vi "AgilentDMM.vi"(4 "error in":T15, 7 "Command":T16) -> (0 "error out":T15, 3 "Response":T13)   [LabVIEW 2018]
uses:
  MOKO_LabViewLibrary/MokoLowLevel/MokoLowLovelControl/MLLC_Command.ctl
  MOKO_LabViewLibrary/MokoLowLevel/MokoLowLovelControl/MLLC_Error.ctl
  MOKO_LabViewLibrary/MokoLowLevel/MokoLowLovelControl/MLLC_Mode.ctl
  MOKO_LabViewLibrary/MokoLowLevel/MokoLowLovelControl/MLLC_Response.ctl
  MOKO_LabViewLibrary/MokoLowLevel/MokoLowLovelControl/MLLC_DriverName.ctl
  MOKO_LabViewLibrary/MokoLowLevel/MokoLowLovelControl/MLLC_Request.ctl
  MOKO_LabViewLibrary/MokoLowLevel/MokoLowLovelControl/MLLC_ErrorCode.ctl
  MOKO_LabViewLibrary/MokoLowLevel/MokoLowLovelControl/MLLC_ResponseInit.ctl
  MOKO_LabViewLibrary/MokoLowLevel/MokoLowLovelControl/MLLC_ConnectCluster.ctl
  MOKO_LabViewLibrary/MokoLowLevel/MokoLowLovelControl/MLLC_InterfaceType.ctl
  MOKO_LabViewLibrary/MokoLowLevel/MokoLowLovelControl/MLLC_OpenedSession.ctl
  MOKO_LabViewLibrary/MokoLowLevel/MokoLowLovelControl/MLLC_InterfaceSettings.ctl
  MOKO_LabViewLibrary/MokoLowLevel/MokoLowLovelControl/MLLC_InterfaceKind.ctl
  data/AgilentDMM_Functions.ctl
  data/AgilentDMM_Models.ctl
panel:
  in  "Settings":T9={"Saved Data"=variant, "Permanent data"={"Connect"={"InterfaceType"=enum."VISA", "OpenedSession"="", "InterfaceSettings"={"Interface"=enum."GPIB", "EOS 4 read"=enum."LF (\\n)", "EOS 4 write"=enum."LF (\\n)", "TMO, ms"=5000, "Sett"=variant(cluster{"Baud Rate":u32, "Data Bits":u16, "Parity":u16, "Stop Bits":u16, "Flow Control":u16, "Eho":bool} {"Baud Rate"=75, "Data Bits"=0, "Parity"=0, "Stop Bits"=0, "Flow Control"=0, "Eho"=FALSE})}}, "Channel"=1, "Func"=enum."VDC", "Model"=enum."L4411"}}
  in  "Response Init array":T10[](array[typedef])=["34401", "34405", "34410", "34411", "34420", "34450", "34461", "34465", "34470", "34475", "U2741"]
  in  "Error Code":T6=5475
  in  "Request":T11="*idn?"
  in  "Driver Name":T12="AgilentDMM"
  in  "Mode":T14=enum."Check"
  # "AgilentDMM"
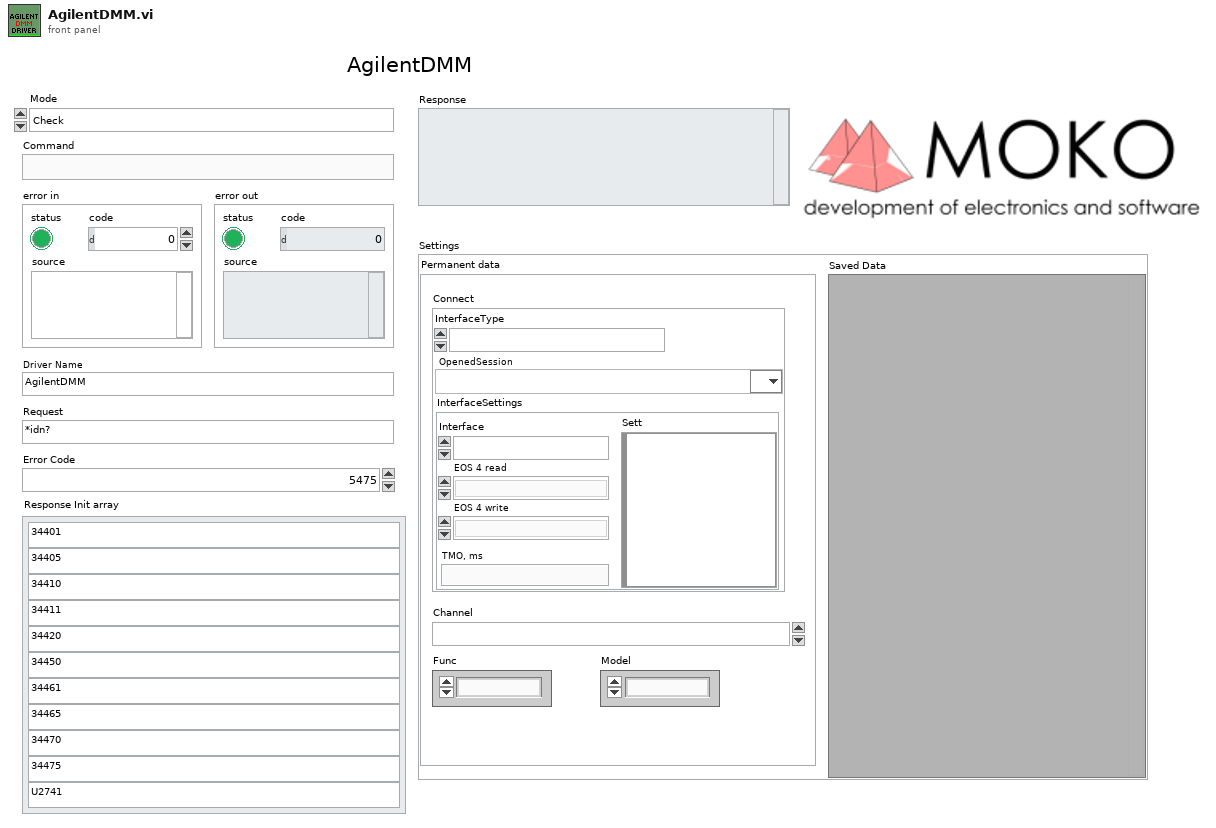
[diagram p1: front panel]
types:
  T1 = typedef "MLLC_ConnectCluster.ctl" = cluster{"InterfaceType":T2, "OpenedSession":T3, "InterfaceSettings":T4}
  T2 = typedef "MLLC_InterfaceType.ctl" = enum16{"VISA", "Prologix USB-GPIB"}
  T3 = typedef "MLLC_OpenedSession.ctl" = refnum<visa-resource-name>
  T4 = typedef "MLLC_InterfaceSettings.ctl" = cluster{"Interface":T5, "EOS 4 read":enum16{"Default (=EOS 4 write)", "CR (\\r)", "LF (\\n)", "None"}, "EOS 4 write":enum16{"CR+LF (\\r\\n)", "CR (\\r)", "LF (\\n)", "None"}, "TMO, ms":i32, "Sett":variant}
  T5 = typedef "MLLC_InterfaceKind.ctl" = enum16{"RS232", "GPIB", "USB", "Ethernet", "another"}
  T6 = typedef "MLLC_ErrorCode.ctl" = u32
  T7 = typedef "AgilentDMM_Functions.ctl" = enum16{"VDC", "VAC", "IDC", "IAC", "F", "R2", "R4", "CAP"}
  T8 = typedef "AgilentDMM_Models.ctl" = enum16{"34401", "34461", "34410", "34411", "34420", "34450", "34405", "U2741", "34470", "34465", "34460", "L4411"}
  T9 = cluster{"Saved Data":variant, "Permanent data":cluster{"Connect":T1, "Channel":T6, "Func":T7, "Model":T8}}
  T10 = typedef "MLLC_ResponseInit.ctl" = string
  T11 = typedef "MLLC_Request.ctl" = string
  T12 = typedef "MLLC_DriverName.ctl" = string
  T13 = typedef "MLLC_Response.ctl" = string
  T14 = typedef "MLLC_Mode.ctl" = enum16{"get", "set", "close", "Init", "Check"}
  T15 = typedef "MLLC_Error.ctl" = errorcluster
  T16 = typedef "MLLC_Command.ctl" = string
  T17 = cluster{"Connect":T1, "Channel":T6, "Func":T7, "Model":T8}
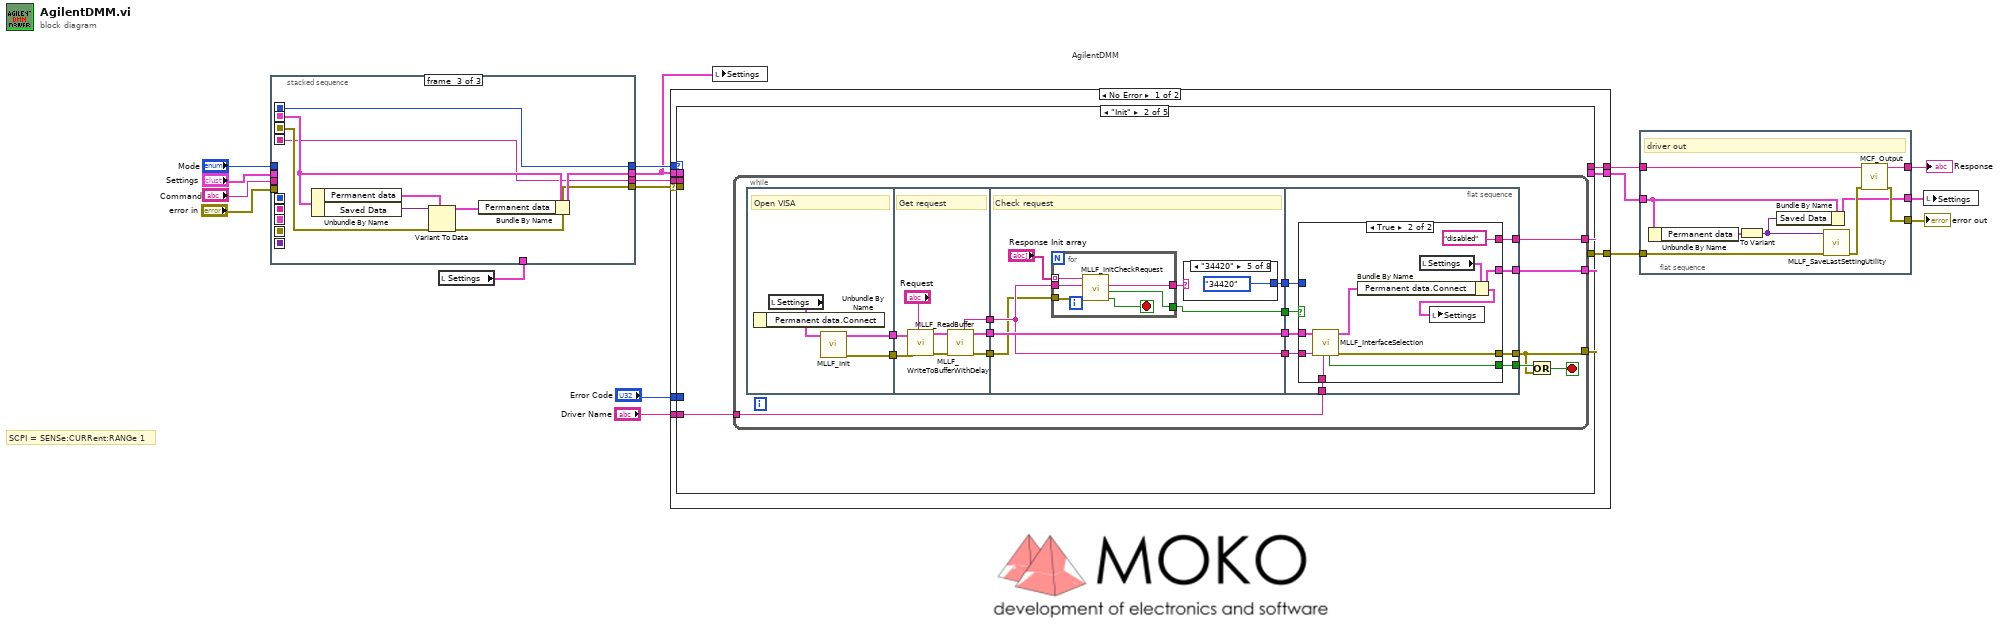
[diagram p0: block diagram]
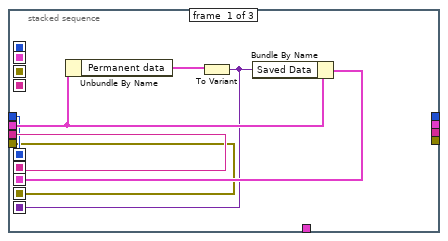
[diagram p2: hidden frame]
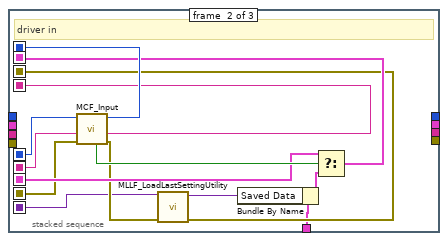
[diagram p3: hidden frame]
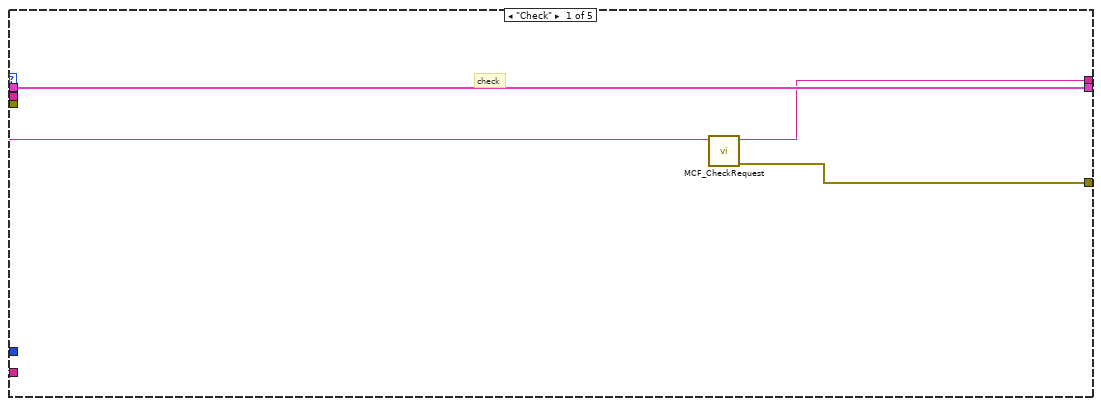
[diagram p4: hidden frame]
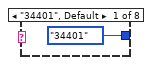
[diagram p5: hidden frame]
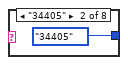
[diagram p6: hidden frame]
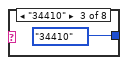
[diagram p7: hidden frame]
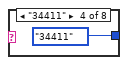
[diagram p8: hidden frame]
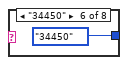
[diagram p9: hidden frame]
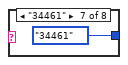
[diagram p10: hidden frame]
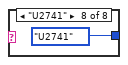
[diagram p11: hidden frame]
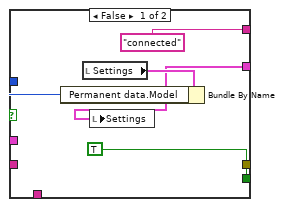
[diagram p12: hidden frame]
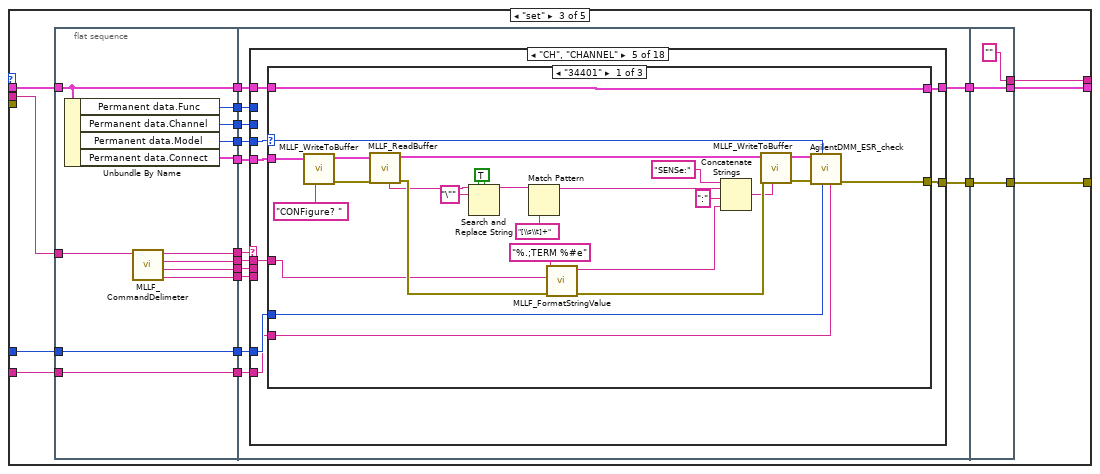
[diagram p13: hidden frame]
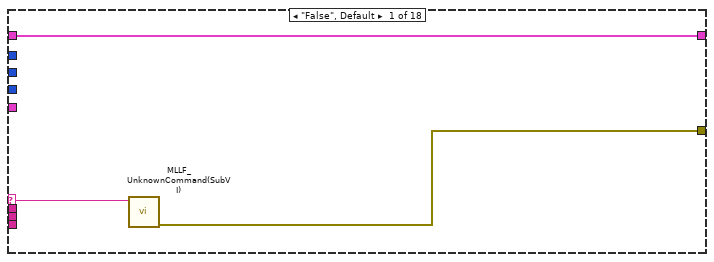
[diagram p14: hidden frame]
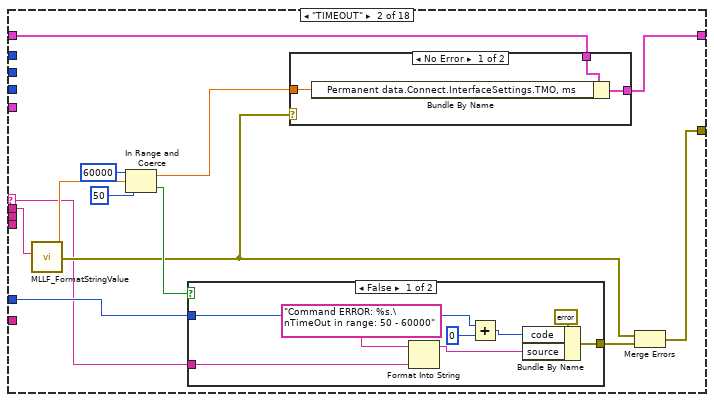
[diagram p15: hidden frame]
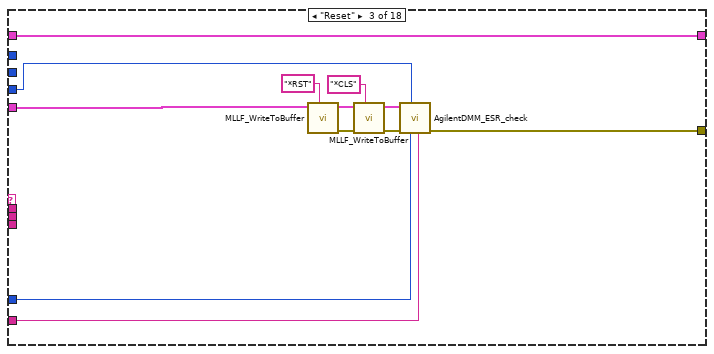
[diagram p18: hidden frame]
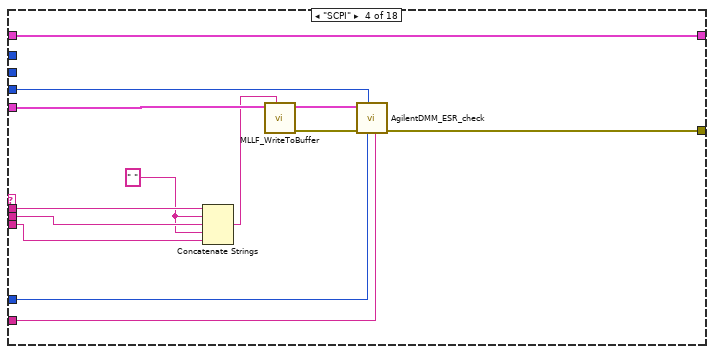
[diagram p19: hidden frame]
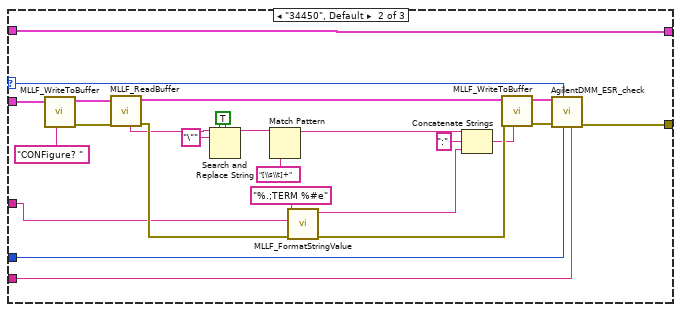
[diagram p20: hidden frame]
diagram:
  # "SCPI = SENSe:CURRent:RANGe 1"
  # "AgilentDMM"
  n1 = local read "Settings"() -> (w8:T9)
  n2 = stacked-sequence {
    seq-local: [w20 _ _] -> [_ w36 _]
    seq-local: [w19 _ _] -> [_ w37 _]
    seq-local: [w22 _ _] -> [_ w32 _]
    seq-local: [w18 _ _] -> [_ w31 _]
    seq-local: [w21 _ _] -> [_ w27 _]
    seq-local: [_ w28 _] -> [_ _ w44]
    seq-local: [_ w38 _] -> [_ _ w41]
    seq-local: [_ w35 _] -> [_ _ w40]
    seq-local: [_ w34 _] -> [_ _ w45]
    tunnel: "Command" -> [w20 _ _]
    tunnel: "Mode" -> [w19 _ _]
    tunnel: "error in" -> [w18 _ _]
    tunnel: "Settings" -> [w23 _ _]
    tunnel: w8 -> [_ w26 _]
    tunnel: [_ _ w40] -> w10
    tunnel: [_ _ w43] -> w1
    tunnel: [_ _ w42] -> w9
    tunnel: [_ _ w41] -> w11
    frame #0 {
      n3 = Unbundle By Name(w23) -> ("Permanent data"=w24:T17)
      n4 = To Variant(anything=w24) -> (Variant=w21:variant)
      n5 = Bundle By Name(cluster=w23, "Saved Data"=w21) -> (w22:T9)
    }
    frame #1 {
      # "driver in"
      n6 = call "MCF_Input.vi"("Error In"=w31, "Command in"=w36, "Mode in"=w37) -> ("Error Out"=w30:errorcluster, "Command out"=w35:string, "Mode out"=w38:T14, "Boolean"=w33:bool)  [unwired: 5 in]
      n7 = call "MLLF_LoadLastSettingUtility.vi"("Error In"=w30, "Save data in"=w27) -> ("Error Out"=w28:errorcluster, "Save data out"=w25:variant)  [unwired: 8 in]
      n8 = Bundle By Name(cluster=w26, "Saved Data"=w25) -> (w29:T9)
      n9 = Select(t=w32, s=w33, f=w29) -> (s? t:f=w34:T9)
    }
    frame #2 {
      n10 = Unbundle By Name(w45) -> ("Permanent data"=w46:T17, "Saved Data"=w39:variant)
      n11 = Variant To Data(error in=w44, type=w46, Variant=w39) -> (data=w47:T17, error out=w42:errorcluster)
      n12 = Bundle By Name(cluster=w45, "Permanent data"=w47) -> (w43:T9)
    }
  }
  n13 = case shown="No Error" w9 {
    selector: w9 -> [w53 w1078]
    tunnel: [w54 w1078] -> w5
    tunnel: w11 -> [w56 _]
    tunnel: [w55 "An error occurred in the driver input module." ("String")] -> w7
    tunnel: w10 -> [w48 _]
    tunnel: w1 -> [w49 w1077]
    tunnel: "Error Code" -> [w52 _]
    tunnel: "Driver Name" -> [w51 _]
    tunnel: [w50 w1077] -> w6
    frame No Error {
      n14 = case shown="\"Init\"" w56 {
        tunnel: [w58 w64 w149 w880 "" ("String")] -> w55
        tunnel: [w59 w62 w152 w881 w1074] -> w54
        tunnel: w53 -> [_ _ _ w898 _]
        tunnel: w52 -> [_ _ w155 w900 _]
        tunnel: w51 -> [w57 w61 w153 w899 _]
        tunnel: [w60 w63 w154 w901 w1073] -> w50
        tunnel: w49 -> [w60 _ w137 w888 w1073]
        tunnel: w48 -> [_ _ w136 w887 _]
        frame "Check" {
          # "check"
          n15 = call "MCF_CheckRequest.vi"("Driver Name"=w57) -> ("Error Out"=w59:errorcluster, "Output String"=w58:string)  [unwired: 9 in]
        }
        frame "Init" {
          n16 = while {
            tunnel: [w67] -> w62
            tunnel: [w66] -> w64
            tunnel: [w65] -> w63
            tunnel: w61 -> [w69]
            stop <- w79 stop-if-true
            n17 = flat-sequence {
              tunnel: [w83] -> w78
              tunnel: [w82] -> w77
              tunnel: w78 -> [w88]
              tunnel: w77 -> [w87]
              tunnel: [w86] -> w76
              tunnel: [w85] -> w75
              tunnel: [w84] -> w74
              tunnel: w76 -> [w94]
              tunnel: w75 -> [w98]
              tunnel: w74 -> [w97]
              tunnel: [w98] -> w73
              tunnel: [w97] -> w72
              tunnel: [w93] -> w71
              tunnel: [w92] -> w70
              tunnel: w73 -> [w120]
              tunnel: w72 -> [w118]
              tunnel: w71 -> [w121]
              tunnel: w70 -> [w119]
              tunnel: w69 -> [w117]
              tunnel: [w116] -> w68
              tunnel: [w115] -> w67
              tunnel: [w114] -> w66
              tunnel: [w113] -> w65
              frame #0 {
                # "Open VISA"
                n18 = local read "Settings"() -> (w81:T9)
                n19 = Unbundle By Name(w81) -> ("Permanent data.Connect"=w80:T1)
                n20 = call "MLLF_Init.vi"("DriverConnect in"=w80) -> ("Error Out"=w83:errorcluster, "DriverConnect out"=w82:T1)  [unwired: 7 in]
              }
              frame #1 {
                # "Get request"
                n21 = call "MLLF_WriteToBufferWithDelay.vi"("Command"="Request", "Error In"=w88, "DriverConnect in"=w87) -> ("Error Out"=w90:errorcluster, "DriverConnect out"=w91:T1)  [unwired: 7 in]
                n22 = call "MLLF_ReadBuffer.vi"("Error In"=w90, "DriverConnect in"=w91) -> ("Error Out"=w86:errorcluster, "DriverConnect out"=w85:T1, "String"=w84:string)  [unwired: 6 in]
              }
              frame #2 {
                # "Check request"
                n23 = for {
                  tunnel: [w101] -> w95
                  tunnel: w97 -> [w103]
                  tunnel: "Response Init array" -> [w104] mode=indexing
                  tunnel: w94 -> [w102]
                  tunnel: [w99] -> w93
                  stop <- w100 stop-if-true
                  n24 = call "MLLF_InitCheckRequest.vi"("error in (no error)"=w102, "Answer"=w103, "Response Init"=w104) -> ("Design ARRAY STOP?"=w100:bool, "Design Interf ARRAY?"=w99:bool, "ResponseInit out"=w101:string)  [unwired: 5 in, 1 out]
                }
                n25 = case shown="\"34420\"" w95 {
                  tunnel: [AgilentDMM_Models."34401" ("Model") AgilentDMM_Models."34405" ("Model") AgilentDMM_Models."34410" ("Model") AgilentDMM_Models."34411" ("Model") AgilentDMM_Models."34420" ("Model") AgilentDMM_Models."34450" ("Model") AgilentDMM_Models."34461" ("Model") AgilentDMM_Models."U2741" ("Model")] -> w92
                  frame "34401", Default {
                  }
                  frame "34405" {
                  }
                  frame "34410" {
                  }
                  frame "34411" {
                  }
                  frame "34420" {
                  }
                  frame "34450" {
                  }
                  frame "34461" {
                  }
                  frame "U2741" {
                  }
                }
              }
              frame #3 {
                n26 = case shown="True" w121 {
                  tunnel: w120 -> [_ w134]
                  tunnel: [TRUE w129] -> w116
                  tunnel: [_ w132] -> w115
                  tunnel: w119 -> [w124 _]
                  tunnel: ["connected" "disabled"] -> w114
                  tunnel: [w122 w130] -> w113
                  tunnel: w118 -> [_ w127]
                  tunnel: w117 -> [_ w128]
                  frame False {
                    n27 = local read "Settings"() -> (w125:T9)
                    n28 = Bundle By Name(cluster=w125, "Permanent data.Model"=w124) -> (w122:T9)
                    n29 = local write "Settings"(w122) -> ()
                  }
                  frame True {
                    n30 = call "MLLF_InterfaceSelection.vi"("Driver Name"=w128, "Answer:"=w127, "DriverConnect in"=w134) -> ("error out"=w132:T15, "DriverConnect out"=w133:T1, "stop init?"=w129:bool)  [unwired: 4 in, 2 out]
                    n31 = local read "Settings"() -> (w135:T9)
                    n32 = Bundle By Name(cluster=w135, "Permanent data.Connect"=w133) -> (w130:T9)
                    n33 = local write "Settings"(w130) -> ()
                  }
                }
              }
            }
            n34 = Or(x=w68, y=w67) -> (x .or. y?=w79:bool)
          }
        }
        frame "set" {
          n35 = flat-sequence {
            tunnel: w153 -> [w166]
            tunnel: w137 -> [w156]
            tunnel: w155 -> [w167]
            tunnel: [w167] -> w148
            tunnel: [w156] -> w147
            tunnel: [w166] -> w146
            tunnel: [w162] -> w145
            tunnel: [w163] -> w144
            tunnel: [w164] -> w143
            tunnel: [w165] -> w142
            tunnel: [w157] -> w141
            tunnel: [w158] -> w140
            tunnel: [w159] -> w139
            tunnel: [w160] -> w138
            tunnel: w136 -> [w161]
            tunnel: [w178] -> w151
            tunnel: [w170] -> w150
            tunnel: w148 -> [w180]
            tunnel: w147 -> [w179]
            tunnel: w146 -> [w177]
            tunnel: w145 -> [w176]
            tunnel: w144 -> [w175]
            tunnel: w143 -> [w174]
            tunnel: w142 -> [w173]
            tunnel: w141 -> [w172]
            tunnel: w140 -> [w171]
            tunnel: w139 -> [w169]
            tunnel: w138 -> [w168]
            tunnel: [w878] -> w152
            tunnel: [w879] -> w154
            tunnel: w151 -> [w879]
            tunnel: w150 -> [w878]
            tunnel: ["" ("String")] -> w149
            frame #0 {
              n36 = Unbundle By Name(w156) -> ("Permanent data.Func"=w165:T7, "Permanent data.Channel"=w164:T6, "Permanent data.Model"=w163:T8, "Permanent data.Connect"=w162:T1)
              n37 = call "MLLF_CommandDelimeter.vi"("command with param"=w161) -> ("param 3"=w160:string, "param 2"=w159:string, "param 1"=w158:string, "command"=w157:string)  [unwired: 6 in, 1 out]
            }
            frame #1 {
              n38 = case shown="\"CH\", \"CHANNEL\"" w172 {
                selector: w172 -> [w182 w185 _ _ _ _ w320 _ _ _ _ _ _ w734 w795 w822 w849 w863]
                tunnel: w171 -> [_ w184 _ w225 w234 _ w321 w396 _ w473 w544 w576 w652 w735 w796 w823 w850 w864]
                tunnel: [w181 w190 w211 w230 w237 _ w327 w400 _ w477 w563 w580 w656 w739 w818 w845 w859 w870] -> w170
                tunnel: w180 -> [_ w191 w213 w232 w240 _ w329 w399 _ w476 w562 w579 w655 w736 w800 w827 w854 w872]
                tunnel: w179 -> [w183 w195 w220 w233 w241 w319 w323 w401 w471 w478 w564 w581 w657 w740 w819 w846 w860 w876]
                tunnel: [w183 w196 w220 w233 w236 w319 w322 w401 w471 w478 w564 w581 w657 w740 w819 w846 w860 w876] -> w178
                tunnel: w176 -> [_ _ w209 w228 w238 _ w326 w397 _ w474 w559 w577 w653 w738 w816 w843 w852 w868]
                tunnel: w177 -> [_ _ w212 w231 w239 _ w328 w398 _ w475 w561 w578 w654 w737 w801 w828 w855 w871]
                tunnel: w175 -> [_ _ w210 w229 w235 _ w325 w395 _ w472 w560 w575 w651 w733 w817 w844 w858 w875]
                tunnel: w174 -> [_ _ _ _ _ _ w324 _ _ _ _ _ _ _ _ _ _ _]
                tunnel: w173 -> [_ _ _ _ _ _ _ _ _ _ _ _ _ _ _ _ _ _]
                tunnel: w169 -> [_ _ _ w224 _ _ _ _ _ _ _ _ _ _ _ _ _ _]
                tunnel: w168 -> [_ _ _ w223 _ _ _ _ _ _ _ _ _ _ _ _ _ _]
                frame "False", Default {
                  n39 = call "MLLF_UnknownCommand(SubVI).vi"("Unknown command"=w182) -> ("error out"=w181:errorcluster)  [unwired: 10 in]
                }
                frame "TIMEOUT" {
                  n40 = call "MLLF_FormatStringValue.vi"("String Value"=w184) -> ("error out"=w186:T15, "number"=w187:dbl)  [unwired: 8 in, 1 out]
                  n41 = In Range and Coerce(upper limit=60000, x=w187, lower limit=50) -> (coerced(x)=w192:dbl, In Range?=w188:bool)
                  n42 = case shown="False" w188 {
                    tunnel: [w203 _] -> w189
                    tunnel: w191 -> [w202 _]
                    tunnel: w185 -> [w201 _]
                    frame False {
                      n43 = Format Into String(format string="Command ERROR: %s.\nTimeOut in range: 50 - 60000", w201) -> (resulting string=w205:string)  [unwired: 2 in, 1 out]
                      n44 = Add(x=w202, y=0) -> (x+y=w206:T6)
                      n45 = Bundle By Name(cluster=errorcluster {"status"=TRUE, "code"=0, "source"=""} ("error out"), "code"=w206, "source"=w205) -> (w203:errorcluster)
                    }
                    frame True {
                    }
                  }
                  n46 = case shown="No Error" w186 {
                    tunnel: [w199 w200] -> w196
                    tunnel: w195 -> [w198 w200]
                    tunnel: w192 -> [w197 _]
                    frame No Error {
                      n47 = Bundle By Name(cluster=w198, "Permanent data.Connect.InterfaceSettings.TMO, ms"=w197) -> (w199:T9)
                    }
                    frame Error {
                    }
                  }
                  n48 = Merge Errors(w186, w189) -> (w190:errorcluster)
                }
                frame "Reset" {
                  n49 = call "MLLF_WriteToBuffer.vi"("String"="*RST", "DriverConnect in"=w209) -> ("error out"=w218:T15, "DriverConnect out"=w219:T1)  [unwired: 6 in]
                  n50 = call "MLLF_WriteToBuffer.vi"("String"="*CLS" ("write buffer"), "error in"=w218, "DriverConnect in"=w219) -> ("error out"=w215:T15, "DriverConnect out"=w214:T1)  [unwired: 5 in]
                  n51 = call "AgilentDMM_ESR_check.vi"("Driver Name"=w212, "Error Code"=w213, "Model"=w210, "error in"=w215, "DriverConnect in"=w214) -> ("error out"=w211:T15)  [unwired: 5 in, 1 out]
                }
                frame "SCPI" {
                  w222 = " " ("string")
                  n52 = Concatenate Strings(w225, w222, w224, w222, w223) -> (w221:string)
                  n53 = call "MLLF_WriteToBuffer.vi"("String"=w221, "DriverConnect in"=w228) -> ("error out"=w226:T15, "DriverConnect out"=w227:T1)  [unwired: 6 in]
                  n54 = call "AgilentDMM_ESR_check.vi"("Driver Name"=w231, "Error Code"=w232, "Model"=w229, "error in"=w226, "DriverConnect in"=w227) -> ("error out"=w230:T15)  [unwired: 5 in, 1 out]
                }
                frame "CH", "CHANNEL" {
                  n55 = case shown="\"34401\"" w235 {
                    selector: w235 -> [w244 w269 w295]
                    tunnel: w241 -> [w246 w271 w300]
                    tunnel: w240 -> [w248 w273 w299]
                    tunnel: w239 -> [w247 w272 w294]
                    tunnel: w238 -> [w245 w270 w298]
                    tunnel: [w249 w274 w297] -> w237
                    tunnel: [w246 w271 w296] -> w236
                    tunnel: w234 -> [w243 w268 w293]
                    frame "34401" {
                      w253 = TRUE ("replace all? (F)")
                      n56 = call "MLLF_WriteToBuffer.vi"("String"="CONFigure? ", "DriverConnect in"=w245) -> ("error out"=w262:T15, "DriverConnect out"=w263:T1)  [unwired: 6 in]
                      n57 = call "MLLF_ReadBuffer.vi"("Error In"=w262, "DriverConnect in"=w263) -> ("Error Out"=w261:errorcluster, "DriverConnect out"=w260:T1, "String"=w255:string)  [unwired: 6 in]
                      n58 = Search and Replace String(replace all?=w253, case sensitive?=w253, input string=w255, search string="\"") -> (result string=w254:string)  [unwired: 4 in, 3 out]
                      n59 = Match Pattern(string=w254, regular expression="[\\s\\t]+") -> (before substring=w256:string)  [unwired: 1 in, 3 out]
                      n60 = call "MLLF_FormatStringValue.vi"("error in"=w261, "String Value"=w243, "Format"="%.;TERM %#e" ("format string")) -> ("error out"=w267:T15, "String Value Formated"=w258:T16)  [unwired: 6 in, 1 out]
                      n61 = Concatenate Strings("SENSe:" ("string"), w256, ":" ("string"), w258) -> (w251:string)
                      n62 = call "MLLF_WriteToBuffer.vi"("String"=w251, "error in"=w267, "DriverConnect in"=w260) -> ("error out"=w266:T15, "DriverConnect out"=w265:T1)  [unwired: 5 in]
                      n63 = call "AgilentDMM_ESR_check.vi"("Driver Name"=w247, "Error Code"=w248, "Model"=w244, "error in"=w266, "DriverConnect in"=w265) -> ("error out"=w249:T15)  [unwired: 5 in, 1 out]
                    }
                    frame "34450", Default {
                      w278 = TRUE ("replace all? (F)")
                      n64 = call "MLLF_WriteToBuffer.vi"("String"="CONFigure? ", "DriverConnect in"=w270) -> ("error out"=w287:T15, "DriverConnect out"=w288:T1)  [unwired: 6 in]
                      n65 = call "MLLF_ReadBuffer.vi"("Error In"=w287, "DriverConnect in"=w288) -> ("Error Out"=w286:errorcluster, "DriverConnect out"=w285:T1, "String"=w280:string)  [unwired: 6 in]
                      n66 = Search and Replace String(replace all?=w278, case sensitive?=w278, input string=w280, search string="\"") -> (result string=w279:string)  [unwired: 4 in, 3 out]
                      n67 = Match Pattern(string=w279, regular expression="[\\s\\t]+") -> (before substring=w281:string)  [unwired: 1 in, 3 out]
                      n68 = call "MLLF_FormatStringValue.vi"("error in"=w286, "String Value"=w268, "Format"="%.;TERM %#e" ("format string")) -> ("error out"=w292:T15, "String Value Formated"=w283:T16)  [unwired: 6 in, 1 out]
                      n69 = Concatenate Strings(w281, ":" ("string"), w283) -> (w276:string)
                      n70 = call "MLLF_WriteToBuffer.vi"("String"=w276, "error in"=w292, "DriverConnect in"=w285) -> ("error out"=w291:T15, "DriverConnect out"=w290:T1)  [unwired: 5 in]
                      n71 = call "AgilentDMM_ESR_check.vi"("Driver Name"=w272, "Error Code"=w273, "Model"=w269, "error in"=w291, "DriverConnect in"=w290) -> ("error out"=w274:T15)  [unwired: 5 in, 1 out]
                    }
                    frame "34420" {
                      n72 = call "MLLF_FormatStringValue.vi"("String Value"=w293, "Format"="%d" ("format")) -> ("error out"=w312:T15, "String Value Formated"=w305:T16)  [unwired: 7 in, 1 out]
                      n73 = call "MLLF_ParameterSelect.vi"("Command to equipment"=string[] ["1", "2"] ("Parameters"), "Names"=string[][] [["1"], ["2"]], "Input"=w305, "Error In"=w312, "Command"=w293, "Driver Name"=w294, "Error Code"=w299) -> ("Choice"=w302:string, "Error Out"=w304:errorcluster)  [unwired: 7 in]
                      n74 = call "MLLF_ParameterSelect.vi"("Command to equipment"=string[] ["ROUTe:TERMinals FRONt1", "ROUTe:TERMinals FRONt2"] ("Names"), "Names"=string[][] [["1"], ["2"]], "Input"=w305, "Error In"=w304, "Command"=w293, "Driver Name"=w294, "Error Code"=w299) -> ("Choice"=w308:string, "Error Out"=w307:errorcluster)  [unwired: 7 in]
                      n75 = call "MLLF_WriteToBuffer.vi"("String"=w308, "error in"=w307, "DriverConnect in"=w298) -> ("error out"=w303:T15, "DriverConnect out"=w306:T1)  [unwired: 5 in]
                      n76 = call "AgilentDMM_ESR_check.vi"("Driver Name"=w294, "Error Code"=w299, "Model"=w295, "error in"=w303, "DriverConnect in"=w306) -> ("error out"=w297:T15)  [unwired: 5 in, 1 out]
                      n77 = Decimal String To Number(string=w302) -> (number=w301:i32)  [unwired: 2 in, 1 out]
                      n78 = case shown="No Error" w297 {
                        tunnel: [w317 w318] -> w296
                        tunnel: w300 -> [w316 w318]
                        tunnel: w301 -> [w315 _]
                        frame No Error {
                          n79 = Bundle By Name(cluster=w316, "Permanent data.Channel"=w315) -> (w317:T9)
                        }
                        frame Error {
                        }
                      }
                    }
                  }
                }
                frame "<----MAIN FUNCTIONS---->" {
                }
                frame "Func", "Function" {
                  # "FUNC=VDC"
                  n80 = case shown="Default" w325 {
                    selector: w325 -> [w356 w378]
                    tunnel: w321 -> [w355 w367]
                    tunnel: w329 -> [w362 w382]
                    tunnel: w328 -> [w361 w381]
                    tunnel: [w360 w380] -> w327
                    tunnel: w326 -> [w358 w379]
                    tunnel: w324 -> [_ w373]
                    tunnel: w320 -> [w354 _]
                    frame Default {
                      n81 = call "MLLF_ParameterSelect.vi"("Command to equipment"=string[] ["CONF:VOLT:DC auto", "CONF:VOLT:AC auto", "CONF:CURR:DC auto", "CONF:CURR:AC auto", "CONF:RES auto", "CONF:FRES auto", "CONF:FREQ", "CONF:TC", "CONF:PER", "CONF:TEMP", "CONF:CAP auto"] ("Names"), "Names"=string[][] [["VDC", "", ""], ["VAC", "", ""], ["IDC", "", ""], ["IAC", "", ""], ["R", "R2", "R2WIRE"], ["R4", "R4WIRE", ""], ["F", "", ""], ["TC", "", ""], ["P", "Period", ""], ["RTD", "PRT", ""], ["C", "CAP", ""]], "Input"=w355, "Command"=w354, "Driver Name"=w361, "Error Code"=w362) -> ("Choice"=w357:string, "Error Out"=w359:errorcluster)  [unwired: 8 in]
                      n82 = call "MLLF_WriteToBuffer.vi"("String"=w357, "error in"=w359, "DriverConnect in"=w358) -> ("error out"=w366:T15, "DriverConnect out"=w365:T1)  [unwired: 5 in]
                      n83 = call "AgilentDMM_ESR_check.vi"("Driver Name"=w361, "Error Code"=w362, "Model"=w356, "error in"=w366, "DriverConnect in"=w365) -> ("error out"=w360:T15)  [unwired: 5 in, 1 out]
                    }
                    frame "34420" {
                      n84 = Equal?(x=u8 1 ("y"), y=w373) -> (x = y?=w375:bool)
                      n85 = Select(t="ROUTe:TERMinals FRONt1" ("String"), s=w375, f="ROUTe:TERMinals FRONt2" ("String")) -> (s? t:f=w369:string)
                      n86 = call "MLLF_ParameterSelect.vi"("Command to equipment"=string[] ["CONF:VOLT:DC auto", "CONF:RES auto", "CONF:FRES auto", "CONF:TC", "CONF:TEMP"] ("Names"), "Names"=string[][] [["VDC", "", ""], ["R", "R2", "R2WIRE"], ["R4", "R4WIRE", ""], ["TC", "", ""], ["RTD", "PRT", ""]], "Input"=w367, "Command"=w367, "Driver Name"=w381, "Error Code"=w382) -> ("Choice"=w368:string, "Error Out"=w370:errorcluster)  [unwired: 8 in]
                      n87 = case shown="\"True\", Default" w368 {
                        selector: w368 -> [w387 w389]
                        tunnel: [w387 w393] -> w372
                        tunnel: [w388 w392] -> w371
                        tunnel: w370 -> [w388 w391]
                        tunnel: w369 -> [_ w390]
                        frame "False" {
                        }
                        frame "True", Default {
                          n88 = Format Into String(format string="%S\n%S", error in=w391, w389, w390) -> (resulting string=w393:string, error out=w392:errorcluster)  [unwired: 1 in]
                        }
                      }
                      n89 = call "MLLF_WriteToBuffer.vi"("String"=w372, "error in"=w371, "DriverConnect in"=w379) -> ("error out"=w386:T15, "DriverConnect out"=w385:T1)  [unwired: 5 in]
                      n90 = call "AgilentDMM_ESR_check.vi"("Driver Name"=w381, "Error Code"=w382, "Model"=w378, "error in"=w386, "DriverConnect in"=w385) -> ("error out"=w380:T15)  [unwired: 5 in, 1 out]
                    }
                  }
                  n91 = case shown="\"IDC\"" w321 {
                    tunnel: w323 -> [w332 w335 w338 w341 w344 w347 w350 w353]
                    tunnel: [w331 w334 w337 w340 w343 w346 w349 w352] -> w322
                    frame "VDC", Default {
                      n92 = Bundle By Name(cluster=w332, "Permanent data.Func"=AgilentDMM_Functions."VDC" ("Func")) -> (w331:T9)
                    }
                    frame "VAC" {
                      n93 = Bundle By Name(cluster=w335, "Permanent data.Func"=AgilentDMM_Functions."VAC" ("Func")) -> (w334:T9)
                    }
                    frame "IDC" {
                      n94 = Bundle By Name(cluster=w338, "Permanent data.Func"=AgilentDMM_Functions."IDC" ("Func")) -> (w337:T9)
                    }
                    frame "IAC" {
                      n95 = Bundle By Name(cluster=w341, "Permanent data.Func"=AgilentDMM_Functions."IAC" ("Func")) -> (w340:T9)
                    }
                    frame "R", "R2", "R2WI" {
                      n96 = Bundle By Name(cluster=w344, "Permanent data.Func"=AgilentDMM_Functions."R2" ("Func")) -> (w343:T9)
                    }
                    frame "R4", "R4WI" {
                      n97 = Bundle By Name(cluster=w347, "Permanent data.Func"=AgilentDMM_Functions."R4" ("Func")) -> (w346:T9)
                    }
                    frame "F" {
                      n98 = Bundle By Name(cluster=w350, "Permanent data.Func"=AgilentDMM_Functions."F" ("Func")) -> (w349:T9)
                    }
                    frame "C", "CAP" {
                      n99 = Bundle By Name(cluster=w353, "Permanent data.Func"=AgilentDMM_Functions."CAP" ("Func")) -> (w352:T9)
                    }
                  }
                }
                frame "Range" {
                  n100 = case shown="\"34401\"" w395 {
                    tunnel: [w421 w456] -> w400
                    tunnel: w399 -> [w420 w455]
                    tunnel: w398 -> [w419 w454]
                    tunnel: w395 -> [w418 w453]
                    tunnel: w397 -> [w417 w452]
                    tunnel: w396 -> [w403 w438]
                    frame "34461", Default {
                      w406 = TRUE ("replace all? (F)")
                      n101 = call "MLLF_WriteToBuffer.vi"("String"="CONFigure? ", "DriverConnect in"=w417) -> ("error out"=w414:T15, "DriverConnect out"=w415:T1)  [unwired: 6 in]
                      n102 = call "MLLF_ReadBuffer.vi"("Error In"=w414, "DriverConnect in"=w415) -> ("Error Out"=w402:errorcluster, "DriverConnect out"=w413:T1, "String"=w408:string)  [unwired: 6 in]
                      n103 = Search and Replace String(replace all?=w406, case sensitive?=w406, input string=w408, search string="\"") -> (result string=w407:string)  [unwired: 4 in, 3 out]
                      n104 = case shown="\"MIN\"" w403 {
                        selector: w403 -> [w426 _ _ _]
                        tunnel: [w429 w430 w432 w434] -> w424
                        tunnel: [w428 "RANG:AUTO ON" ("String") "RANG MIN" ("String") "RANG MAX" ("String")] -> w411
                        tunnel: w402 -> [w425 w430 w432 w434]
                        frame "False", Default {
                          n105 = call "MLLF_FormatStringValue.vi"("error in"=w425, "String Value"=w426, "Format"="RANG %#e" ("format string")) -> ("error out"=w429:T15, "String Value Formated"=w428:T16)  [unwired: 6 in, 1 out]
                        }
                        frame "Auto" {
                        }
                        frame "MIN" {
                        }
                        frame "MAX" {
                        }
                      }
                      n106 = Match Pattern(string=w407, regular expression="[\\s\\t]+") -> (before substring=w409:string)  [unwired: 1 in, 3 out]
                      n107 = Concatenate Strings(w409, ":" ("string"), w411) -> (w404:string)
                      n108 = call "MLLF_WriteToBuffer.vi"("String"=w404, "error in"=w424, "DriverConnect in"=w413) -> ("error out"=w423:T15, "DriverConnect out"=w422:T1)  [unwired: 5 in]
                      n109 = call "AgilentDMM_ESR_check.vi"("Driver Name"=w419, "Error Code"=w420, "Model"=w418, "error in"=w423, "DriverConnect in"=w422) -> ("error out"=w421:T15)  [unwired: 5 in, 1 out]
                    }
                    frame "34401" {
                      w441 = TRUE ("replace all? (F)")
                      n110 = call "MLLF_WriteToBuffer.vi"("String"="CONFigure? ", "DriverConnect in"=w452) -> ("error out"=w449:T15, "DriverConnect out"=w450:T1)  [unwired: 6 in]
                      n111 = call "MLLF_ReadBuffer.vi"("Error In"=w449, "DriverConnect in"=w450) -> ("Error Out"=w437:errorcluster, "DriverConnect out"=w448:T1, "String"=w443:string)  [unwired: 6 in]
                      n112 = Search and Replace String(replace all?=w441, case sensitive?=w441, input string=w443, search string="\"") -> (result string=w442:string)  [unwired: 4 in, 3 out]
                      n113 = case shown="\"MIN\"" w438 {
                        selector: w438 -> [w461 _ _ _]
                        tunnel: [w464 w465 w467 w469] -> w459
                        tunnel: [w463 "RANG:AUTO ON" ("String") "RANG MIN" ("String") "RANG MAX" ("String")] -> w446
                        tunnel: w437 -> [w460 w465 w467 w469]
                        frame "False", Default {
                          n114 = call "MLLF_FormatStringValue.vi"("error in"=w460, "String Value"=w461, "Format"="RANG %#e" ("format string")) -> ("error out"=w464:T15, "String Value Formated"=w463:T16)  [unwired: 6 in, 1 out]
                        }
                        frame "Auto" {
                        }
                        frame "MIN" {
                        }
                        frame "MAX" {
                        }
                      }
                      n115 = Match Pattern(string=w442, regular expression="[\\s\\t]+") -> (before substring=w444:string)  [unwired: 1 in, 3 out]
                      n116 = Concatenate Strings("SENSe:" ("string"), w444, ":" ("string"), w446) -> (w439:string)
                      n117 = call "MLLF_WriteToBuffer.vi"("String"=w439, "error in"=w459, "DriverConnect in"=w448) -> ("error out"=w458:T15, "DriverConnect out"=w457:T1)  [unwired: 5 in]
                      n118 = call "AgilentDMM_ESR_check.vi"("Driver Name"=w454, "Error Code"=w455, "Model"=w453, "error in"=w458, "DriverConnect in"=w457) -> ("error out"=w456:T15)  [unwired: 5 in, 1 out]
                    }
                  }
                }
                frame "---------ADDITIONAL---------" {
                }
                frame "Res", "Resolution" {
                  n119 = case shown="\"34401\"" w472 {
                    selector: w472 -> [w479 w512]
                    tunnel: [w498 w531] -> w477
                    tunnel: w476 -> [w497 w530]
                    tunnel: w475 -> [w496 w529]
                    tunnel: w474 -> [w495 w528]
                    tunnel: w473 -> [w480 w513]
                    frame "34461", Default {
                      w483 = TRUE ("replace all? (F)")
                      n120 = call "MLLF_WriteToBuffer.vi"("String"="CONFigure? ", "DriverConnect in"=w495) -> ("error out"=w492:T15, "DriverConnect out"=w493:T1)  [unwired: 6 in]
                      n121 = call "MLLF_ReadBuffer.vi"("Error In"=w492, "DriverConnect in"=w493) -> ("Error Out"=w491:errorcluster, "DriverConnect out"=w490:T1, "String"=w485:string)  [unwired: 6 in]
                      n122 = Search and Replace String(replace all?=w483, case sensitive?=w483, input string=w485, search string="\"") -> (result string=w484:string)  [unwired: 4 in, 3 out]
                      n123 = case shown="\"MAX\"" w480 {
                        selector: w480 -> [w503 _ _]
                        tunnel: [w506 w507 w509] -> w501
                        tunnel: [w505 "RES MAX" ("String") "RES MIN" ("String")] -> w488
                        tunnel: w491 -> [w502 w507 w509]
                        frame "False", Default {
                          n124 = call "MLLF_FormatStringValue.vi"("error in"=w502, "String Value"=w503, "Format"="RES %#e" ("format string")) -> ("error out"=w506:T15, "String Value Formated"=w505:T16)  [unwired: 6 in, 1 out]
                        }
                        frame "MAX" {
                        }
                        frame "MIN" {
                        }
                      }
                      n125 = Match Pattern(string=w484, regular expression="[\\s\\t]+") -> (before substring=w486:string)  [unwired: 1 in, 3 out]
                      n126 = Concatenate Strings(w486, ":" ("string"), w488) -> (w481:string)
                      n127 = call "MLLF_WriteToBuffer.vi"("String"=w481, "error in"=w501, "DriverConnect in"=w490) -> ("error out"=w500:T15, "DriverConnect out"=w499:T1)  [unwired: 5 in]
                      n128 = call "AgilentDMM_ESR_check.vi"("Driver Name"=w496, "Error Code"=w497, "Model"=w479, "error in"=w500, "DriverConnect in"=w499) -> ("error out"=w498:T15)  [unwired: 5 in, 1 out]
                    }
                    frame "34401" {
                      w516 = TRUE ("replace all? (F)")
                      n129 = call "MLLF_WriteToBuffer.vi"("String"="CONFigure? ", "DriverConnect in"=w528) -> ("error out"=w525:T15, "DriverConnect out"=w526:T1)  [unwired: 6 in]
                      n130 = call "MLLF_ReadBuffer.vi"("Error In"=w525, "DriverConnect in"=w526) -> ("Error Out"=w524:errorcluster, "DriverConnect out"=w523:T1, "String"=w518:string)  [unwired: 6 in]
                      n131 = Search and Replace String(replace all?=w516, case sensitive?=w516, input string=w518, search string="\"") -> (result string=w517:string)  [unwired: 4 in, 3 out]
                      n132 = case shown="\"MIN\"" w513 {
                        selector: w513 -> [w536 _ _]
                        tunnel: [w539 w540 w542] -> w534
                        tunnel: [w538 "RES MAX" ("String") "RES MIN" ("String")] -> w521
                        tunnel: w524 -> [w535 w540 w542]
                        frame "False", Default {
                          n133 = call "MLLF_FormatStringValue.vi"("error in"=w535, "String Value"=w536, "Format"="RES %#e" ("format string")) -> ("error out"=w539:T15, "String Value Formated"=w538:T16)  [unwired: 6 in, 1 out]
                        }
                        frame "MAX" {
                        }
                        frame "MIN" {
                        }
                      }
                      n134 = Match Pattern(string=w517, regular expression="[\\s\\t]+") -> (before substring=w519:string)  [unwired: 1 in, 3 out]
                      n135 = Concatenate Strings("SENSe:" ("string"), w519, ":" ("string"), w521) -> (w514:string)
                      n136 = call "MLLF_WriteToBuffer.vi"("String"=w514, "error in"=w534, "DriverConnect in"=w523) -> ("error out"=w533:T15, "DriverConnect out"=w532:T1)  [unwired: 5 in]
                      n137 = call "AgilentDMM_ESR_check.vi"("Driver Name"=w529, "Error Code"=w530, "Model"=w512, "error in"=w533, "DriverConnect in"=w532) -> ("error out"=w531:T15)  [unwired: 5 in, 1 out]
                    }
                  }
                }
                frame "Aper", "Aperture", "MeasTime" {
                  w547 = TRUE ("replace all? (F)")
                  n138 = call "MLLF_WriteToBuffer.vi"("String"="CONFigure? ", "DriverConnect in"=w559) -> ("error out"=w556:T15, "DriverConnect out"=w557:T1)  [unwired: 6 in]
                  n139 = call "MLLF_ReadBuffer.vi"("Error In"=w556, "DriverConnect in"=w557) -> ("Error Out"=w555:errorcluster, "DriverConnect out"=w554:T1, "String"=w549:string)  [unwired: 6 in]
                  n140 = Search and Replace String(replace all?=w547, case sensitive?=w547, input string=w549, search string="\"") -> (result string=w548:string)  [unwired: 4 in, 3 out]
                  n141 = case shown="\"OFF\"" w544 {
                    selector: w544 -> [w569 _]
                    tunnel: [w572 w573] -> w567
                    tunnel: [w571 "APER:ENAB OFF" ("String")] -> w552
                    tunnel: w555 -> [w568 w573]
                    frame "False", Default {
                      n142 = call "MLLF_FormatStringValue.vi"("error in"=w568, "String Value"=w569, "Format"="APER %#e" ("format string")) -> ("error out"=w572:T15, "String Value Formated"=w571:T16)  [unwired: 6 in, 1 out]
                    }
                    frame "OFF" {
                    }
                  }
                  n143 = Match Pattern(string=w548, regular expression="[\\s\\t]+") -> (before substring=w550:string)  [unwired: 1 in, 3 out]
                  n144 = Concatenate Strings(w550, ":" ("string"), w552) -> (w545:string)
                  n145 = call "MLLF_WriteToBuffer.vi"("String"=w545, "error in"=w567, "DriverConnect in"=w554) -> ("error out"=w566:T15, "DriverConnect out"=w565:T1)  [unwired: 5 in]
                  n146 = call "AgilentDMM_ESR_check.vi"("Driver Name"=w561, "Error Code"=w562, "Model"=w560, "error in"=w566, "DriverConnect in"=w565) -> ("error out"=w563:T15)  [unwired: 5 in, 1 out]
                }
                frame "IntegrationTime", "IntTime", "NPLC" {
                  n147 = case shown="\"34401\"" w575 {
                    tunnel: [w601 w635] -> w580
                    tunnel: w579 -> [w600 w634]
                    tunnel: w578 -> [w599 w633]
                    tunnel: w575 -> [w598 w632]
                    tunnel: w577 -> [w597 w631]
                    tunnel: w576 -> [w583 w617]
                    frame "34401" {
                      w586 = TRUE ("replace all? (F)")
                      n148 = call "MLLF_WriteToBuffer.vi"("String"="CONFigure? ", "DriverConnect in"=w597) -> ("error out"=w594:T15, "DriverConnect out"=w595:T1)  [unwired: 6 in]
                      n149 = call "MLLF_ReadBuffer.vi"("Error In"=w594, "DriverConnect in"=w595) -> ("DriverConnect out"=w593:T1, "String"=w588:string)  [unwired: 6 in, 1 out]
                      n150 = Search and Replace String(replace all?=w586, case sensitive?=w586, input string=w588, search string="\"") -> (result string=w587:string)  [unwired: 4 in, 3 out]
                      n151 = case shown="\"MIN\"" w583 {
                        tunnel: [w608 w612 w616] -> w604
                        tunnel: [w607 w611 w615] -> w591
                        tunnel: w583 -> [w605 w609 w613]
                        frame Default {
                          n152 = call "MLLF_FormatStringValue.vi"("String Value"=w605, "Format"="NPLC %#e" ("format string")) -> ("error out"=w608:T15, "String Value Formated"=w607:T16)  [unwired: 7 in, 1 out]
                        }
                        frame "MIN" {
                          n153 = call "MLLF_FormatStringValue.vi"("String Value"=w609, "Format"="NPLC MIN" ("format string")) -> ("error out"=w612:T15, "String Value Formated"=w611:T16)  [unwired: 7 in, 1 out]
                        }
                        frame "MAX" {
                          n154 = call "MLLF_FormatStringValue.vi"("String Value"=w613, "Format"="NPLC MAX" ("format string")) -> ("error out"=w616:T15, "String Value Formated"=w615:T16)  [unwired: 7 in, 1 out]
                        }
                      }
                      n155 = Match Pattern(string=w587, regular expression="[\\s\\t]+") -> (before substring=w589:string)  [unwired: 1 in, 3 out]
                      n156 = Concatenate Strings("SENSe:" ("string"), w589, ":" ("string"), w591) -> (w584:string)
                      n157 = call "MLLF_WriteToBuffer.vi"("String"=w584, "error in"=w604, "DriverConnect in"=w593) -> ("error out"=w603:T15, "DriverConnect out"=w602:T1)  [unwired: 5 in]
                      n158 = call "AgilentDMM_ESR_check.vi"("Driver Name"=w599, "Error Code"=w600, "Model"=w598, "error in"=w603, "DriverConnect in"=w602) -> ("error out"=w601:T15)  [unwired: 5 in, 1 out]
                    }
                    frame Default {
                      w620 = TRUE ("replace all? (F)")
                      n159 = call "MLLF_WriteToBuffer.vi"("String"="CONFigure? ", "DriverConnect in"=w631) -> ("error out"=w628:T15, "DriverConnect out"=w629:T1)  [unwired: 6 in]
                      n160 = call "MLLF_ReadBuffer.vi"("Error In"=w628, "DriverConnect in"=w629) -> ("DriverConnect out"=w627:T1, "String"=w622:string)  [unwired: 6 in, 1 out]
                      n161 = Search and Replace String(replace all?=w620, case sensitive?=w620, input string=w622, search string="\"") -> (result string=w621:string)  [unwired: 4 in, 3 out]
                      n162 = case shown="Default" w617 {
                        tunnel: [w642 w646 w650] -> w638
                        tunnel: [w641 w645 w649] -> w625
                        tunnel: w617 -> [w639 w643 w647]
                        frame Default {
                          n163 = call "MLLF_FormatStringValue.vi"("String Value"=w639, "Format"="%.;NPLC %#e" ("format string")) -> ("error out"=w642:T15, "String Value Formated"=w641:T16)  [unwired: 7 in, 1 out]
                        }
                        frame "MIN" {
                          n164 = call "MLLF_FormatStringValue.vi"("String Value"=w643, "Format"="NPLC MIN" ("format string")) -> ("error out"=w646:T15, "String Value Formated"=w645:T16)  [unwired: 7 in, 1 out]
                        }
                        frame "MAX" {
                          n165 = call "MLLF_FormatStringValue.vi"("String Value"=w647, "Format"="NPLC MAX" ("format string")) -> ("error out"=w650:T15, "String Value Formated"=w649:T16)  [unwired: 7 in, 1 out]
                        }
                      }
                      n166 = Match Pattern(string=w621, regular expression="[\\s\\t]+") -> (before substring=w623:string)  [unwired: 1 in, 3 out]
                      n167 = Concatenate Strings(w623, ":" ("string"), w625) -> (w618:string)
                      n168 = call "MLLF_WriteToBuffer.vi"("String"=w618, "error in"=w638, "DriverConnect in"=w627) -> ("error out"=w637:T15, "DriverConnect out"=w636:T1)  [unwired: 5 in]
                      n169 = call "AgilentDMM_ESR_check.vi"("Driver Name"=w633, "Error Code"=w634, "Model"=w632, "error in"=w637, "DriverConnect in"=w636) -> ("error out"=w635:T15)  [unwired: 5 in, 1 out]
                    }
                  }
                }
                frame "ACBand", "ACBandwidth", "Band", "Bandwidth" {
                  n170 = case shown="\"34401\"" w651 {
                    selector: w651 -> [w658 w696]
                    tunnel: [w677 w714] -> w656
                    tunnel: w655 -> [w676 w713]
                    tunnel: w654 -> [w675 w712]
                    tunnel: w653 -> [w674 w711]
                    tunnel: w652 -> [w659 w698]
                    frame "34461", Default {
                      w662 = TRUE ("replace all? (F)")
                      n171 = call "MLLF_WriteToBuffer.vi"("String"="CONFigure? ", "DriverConnect in"=w674) -> ("error out"=w671:T15, "DriverConnect out"=w672:T1)  [unwired: 6 in]
                      n172 = call "MLLF_ReadBuffer.vi"("Error In"=w671, "DriverConnect in"=w672) -> ("Error Out"=w670:errorcluster, "DriverConnect out"=w669:T1, "String"=w664:string)  [unwired: 6 in]
                      n173 = case shown="\"MIN\"" w659 {
                        selector: w659 -> [w681 w686 w691]
                        tunnel: [w685 w690 w695] -> w680
                        tunnel: w670 -> [w684 w689 w694]
                        tunnel: [w683 w688 w693] -> w667
                        frame Default {
                          n174 = call "MLLF_FormatStringValue.vi"("error in"=w684, "String Value"=w681, "Format"="%.;BAND %#f" ("format string")) -> ("error out"=w685:T15, "String Value Formated"=w683:T16)  [unwired: 6 in, 1 out]
                        }
                        frame "MAX" {
                          n175 = call "MLLF_FormatStringValue.vi"("error in"=w689, "String Value"=w686, "Format"="BAND MAX" ("format string")) -> ("error out"=w690:T15, "String Value Formated"=w688:T16)  [unwired: 6 in, 1 out]
                        }
                        frame "MIN" {
                          n176 = call "MLLF_FormatStringValue.vi"("error in"=w694, "String Value"=w691, "Format"="BAND MIN" ("format string")) -> ("error out"=w695:T15, "String Value Formated"=w693:T16)  [unwired: 6 in, 1 out]
                        }
                      }
                      n177 = Search and Replace String(replace all?=w662, case sensitive?=w662, input string=w664, search string="\"") -> (result string=w663:string)  [unwired: 4 in, 3 out]
                      n178 = Match Pattern(string=w663, regular expression="[\\s\\t]+") -> (before substring=w665:string)  [unwired: 1 in, 3 out]
                      n179 = Concatenate Strings(w665, ":" ("string"), w667) -> (w660:string)
                      n180 = call "MLLF_WriteToBuffer.vi"("String"=w660, "error in"=w680, "DriverConnect in"=w669) -> ("error out"=w679:T15, "DriverConnect out"=w678:T1)  [unwired: 5 in]
                      n181 = call "AgilentDMM_ESR_check.vi"("Driver Name"=w675, "Error Code"=w676, "Model"=w658, "error in"=w679, "DriverConnect in"=w678) -> ("error out"=w677:T15)  [unwired: 5 in, 1 out]
                    }
                    frame "34401" {
                      w701 = TRUE ("replace all? (F)")
                      n182 = call "MLLF_WriteToBuffer.vi"("String"="CONFigure? ", "DriverConnect in"=w711) -> ("error out"=w708:T15, "DriverConnect out"=w709:T1)  [unwired: 6 in]
                      n183 = call "MLLF_ReadBuffer.vi"("Error In"=w708, "DriverConnect in"=w709) -> ("Error Out"=w707:errorcluster, "DriverConnect out"=w706:T1, "String"=w703:string)  [unwired: 6 in]
                      n184 = case shown="\"MAX\"" w698 {
                        tunnel: [w722 w727 w732] -> w717
                        tunnel: w707 -> [w721 w726 w731]
                        tunnel: [w720 w725 w730] -> w704
                        tunnel: w698 -> [w718 w723 w728]
                        frame Default {
                          n185 = call "MLLF_FormatStringValue.vi"("error in"=w721, "String Value"=w718, "Format"="BAND %#f" ("format string")) -> ("error out"=w722:T15, "String Value Formated"=w720:T16)  [unwired: 6 in, 1 out]
                        }
                        frame "MAX" {
                          n186 = call "MLLF_FormatStringValue.vi"("error in"=w726, "String Value"=w723, "Format"="BAND MAX" ("format string")) -> ("error out"=w727:T15, "String Value Formated"=w725:T16)  [unwired: 6 in, 1 out]
                        }
                        frame "MIN" {
                          n187 = call "MLLF_FormatStringValue.vi"("error in"=w731, "String Value"=w728, "Format"="BAND MIN" ("format string")) -> ("error out"=w732:T15, "String Value Formated"=w730:T16)  [unwired: 6 in, 1 out]
                        }
                      }
                      n188 = Search and Replace String(replace all?=w701, case sensitive?=w701, input string=w703, search string="\"") -> (result string=w702:string)  [unwired: 4 in, 3 out]
                      n189 = Match Pattern(string=w702, regular expression="[\\s\\t]+") -> ()  [unwired: 1 in, 4 out]
                      n190 = Concatenate Strings(":DET:" ("string"), w704) -> (w699:string)
                      n191 = call "MLLF_WriteToBuffer.vi"("String"=w699, "error in"=w717, "DriverConnect in"=w706) -> ("error out"=w716:T15, "DriverConnect out"=w715:T1)  [unwired: 5 in]
                      n192 = call "AgilentDMM_ESR_check.vi"("Driver Name"=w712, "Error Code"=w713, "Model"=w696, "error in"=w716, "DriverConnect in"=w715) -> ("error out"=w714:T15)  [unwired: 5 in, 1 out]
                    }
                  }
                }
                frame "AutoZero", "ZERO" {
                  n193 = case shown="\"34461\", Default" w733 {
                    tunnel: [w764 w792] -> w739
                    tunnel: w733 -> [w763 w791]
                    tunnel: w738 -> [w762 w790]
                    tunnel: w737 -> [w747 w775]
                    tunnel: w736 -> [w746 w774]
                    tunnel: w735 -> [w742 w770]
                    tunnel: w734 -> [w741 w769]
                    frame "34461", Default {
                      w752 = TRUE ("replace all? (F)")
                      n194 = call "MLLF_WriteToBuffer.vi"("String"="CONFigure? ", "DriverConnect in"=w762) -> ("error out"=w759:T15, "DriverConnect out"=w760:T1)  [unwired: 6 in]
                      n195 = call "MLLF_ReadBuffer.vi"("Error In"=w759, "DriverConnect in"=w760) -> ("Error Out"=w744:errorcluster, "DriverConnect out"=w758:T1, "String"=w754:string)  [unwired: 6 in]
                      n196 = Search and Replace String(replace all?=w752, case sensitive?=w752, input string=w754, search string="\"") -> (result string=w753:string)  [unwired: 4 in, 3 out]
                      n197 = Match Pattern(string=w753, regular expression="[\\s\\t]+") -> (before substring=w755:string)  [unwired: 1 in, 3 out]
                      n198 = call "MLLF_ParameterSelect.vi"("Command to equipment"=string[] ["ZERO:AUTO OFF", "ZERO:AUTO ON", "ZERO:AUTO ONCE"] ("Names"), "Names"=string[][] [["0", "DIS", "DISABLE", "DISABLED", "OFF"], ["1", "EN", "ENABLE", "ENABLED", "ON"], [" ", "", "", "", ""]], "Input"=w742, "Error In"=w744, "Command"=w741, "Driver Name"=w747, "Error Code"=w746) -> ("Choice"=w743:string, "Error Out"=w745:errorcluster)  [unwired: 7 in]
                      n199 = Concatenate Strings(w755, ":" ("string"), w743) -> (w750:string)
                      n200 = call "MLLF_WriteToBuffer.vi"("String"=w750, "error in"=w745, "DriverConnect in"=w758) -> ("error out"=w766:T15, "DriverConnect out"=w765:T1)  [unwired: 5 in]
                      n201 = call "AgilentDMM_ESR_check.vi"("Driver Name"=w747, "Error Code"=w746, "Model"=w763, "error in"=w766, "DriverConnect in"=w765) -> ("error out"=w764:T15)  [unwired: 5 in, 1 out]
                    }
                    frame "34401" {
                      w780 = TRUE ("replace all? (F)")
                      n202 = call "MLLF_WriteToBuffer.vi"("String"="CONFigure? ", "DriverConnect in"=w790) -> ("error out"=w787:T15, "DriverConnect out"=w788:T1)  [unwired: 6 in]
                      n203 = call "MLLF_ReadBuffer.vi"("Error In"=w787, "DriverConnect in"=w788) -> ("Error Out"=w772:errorcluster, "DriverConnect out"=w786:T1, "String"=w782:string)  [unwired: 6 in]
                      n204 = Search and Replace String(replace all?=w780, case sensitive?=w780, input string=w782, search string="\"") -> (result string=w781:string)  [unwired: 4 in, 3 out]
                      n205 = Match Pattern(string=w781, regular expression="[\\s\\t]+") -> (before substring=w783:string)  [unwired: 1 in, 3 out]
                      n206 = call "MLLF_ParameterSelect.vi"("Command to equipment"=string[] ["ZERO:AUTO OFF", "ZERO:AUTO ON", "ZERO:AUTO ONCE"] ("Names"), "Ignor case(default = true)"=TRUE, "Names"=string[][] [["OFF"], ["ON"], ["ONCE"]], "Input"=w770, "Error In"=w772, "Command"=w769, "Driver Name"=w775, "Error Code"=w774) -> ("Choice"=w771:string, "Error Out"=w773:errorcluster)  [unwired: 6 in]
                      n207 = Concatenate Strings("SENSe:" ("string"), w783, ":" ("string"), w771) -> (w778:string)
                      n208 = call "MLLF_WriteToBuffer.vi"("String"=w778, "error in"=w773, "DriverConnect in"=w786) -> ("error out"=w794:T15, "DriverConnect out"=w793:T1)  [unwired: 5 in]
                      n209 = call "AgilentDMM_ESR_check.vi"("Driver Name"=w775, "Error Code"=w774, "Model"=w791, "error in"=w794, "DriverConnect in"=w793) -> ("error out"=w792:T15)  [unwired: 5 in, 1 out]
                    }
                  }
                }
                frame "LOWPOWER" {
                  w806 = TRUE ("replace all? (F)")
                  n210 = call "MLLF_WriteToBuffer.vi"("String"="CONFigure? ", "DriverConnect in"=w816) -> ("error out"=w813:T15, "DriverConnect out"=w814:T1)  [unwired: 6 in]
                  n211 = call "MLLF_ReadBuffer.vi"("Error In"=w813, "DriverConnect in"=w814) -> ("Error Out"=w798:errorcluster, "DriverConnect out"=w812:T1, "String"=w808:string)  [unwired: 6 in]
                  n212 = Search and Replace String(replace all?=w806, case sensitive?=w806, input string=w808, search string="\"") -> (result string=w807:string)  [unwired: 4 in, 3 out]
                  n213 = Match Pattern(string=w807, regular expression="[\\s\\t]+") -> (before substring=w809:string)  [unwired: 1 in, 3 out]
                  n214 = call "MLLF_ParameterSelect.vi"("Command to equipment"=string[] ["POW:LIM OFF", "POW:LIM ON"] ("Names"), "Names"=string[][] [["0", "DIS", "DISABLE", "DISABLED", "OFF"], ["1", "EN", "ENABLE", "ENABLED", "ON"]], "Input"=w796, "Error In"=w798, "Command"=w795, "Driver Name"=w801, "Error Code"=w800) -> ("Choice"=w797:string, "Error Out"=w799:errorcluster)  [unwired: 7 in]
                  n215 = Concatenate Strings(w809, ":" ("string"), w797) -> (w804:string)
                  n216 = call "MLLF_WriteToBuffer.vi"("String"=w804, "error in"=w799, "DriverConnect in"=w812) -> ("error out"=w821:T15, "DriverConnect out"=w820:T1)  [unwired: 5 in]
                  n217 = call "AgilentDMM_ESR_check.vi"("Driver Name"=w801, "Error Code"=w800, "Model"=w817, "error in"=w821, "DriverConnect in"=w820) -> ("error out"=w818:T15)  [unwired: 5 in, 1 out]
                }
                frame "VOLTAGELIMITED" {
                  w833 = TRUE ("replace all? (F)")
                  n218 = call "MLLF_WriteToBuffer.vi"("String"="CONFigure? ", "DriverConnect in"=w843) -> ("error out"=w840:T15, "DriverConnect out"=w841:T1)  [unwired: 6 in]
                  n219 = call "MLLF_ReadBuffer.vi"("Error In"=w840, "DriverConnect in"=w841) -> ("Error Out"=w825:errorcluster, "DriverConnect out"=w839:T1, "String"=w835:string)  [unwired: 6 in]
                  n220 = Search and Replace String(replace all?=w833, case sensitive?=w833, input string=w835, search string="\"") -> (result string=w834:string)  [unwired: 4 in, 3 out]
                  n221 = Match Pattern(string=w834, regular expression="[\\s\\t]+") -> (before substring=w836:string)  [unwired: 1 in, 3 out]
                  n222 = call "MLLF_ParameterSelect.vi"("Command to equipment"=string[] ["VOLT:LIM OFF", "VOLT:LIM ON"] ("Names"), "Names"=string[][] [["0", "DIS", "DISABLE", "DISABLED", "OFF"], ["1", "EN", "ENABLE", "ENABLED", "ON"]], "Input"=w823, "Error In"=w825, "Command"=w822, "Driver Name"=w828, "Error Code"=w827) -> ("Choice"=w824:string, "Error Out"=w826:errorcluster)  [unwired: 7 in]
                  n223 = Concatenate Strings(w836, ":" ("string"), w824) -> (w831:string)
                  n224 = call "MLLF_WriteToBuffer.vi"("String"=w831, "error in"=w826, "DriverConnect in"=w839) -> ("error out"=w848:T15, "DriverConnect out"=w847:T1)  [unwired: 5 in]
                  n225 = call "AgilentDMM_ESR_check.vi"("Driver Name"=w828, "Error Code"=w827, "Model"=w844, "error in"=w848, "DriverConnect in"=w847) -> ("error out"=w845:T15)  [unwired: 5 in, 1 out]
                }
                frame "FILT", "FILTER" {
                  # "FILT=DIS"
                  n226 = call "MLLF_ParameterSelect.vi"("Command to equipment"=string[] ["INPut:FILTer:STATE OFF", "INPut:FILTer:STATE ON"] ("Names"), "Names"=string[][] [["0", "DIS", "DISABLE", "DISABLED", "OFF"], ["1", "EN", "ENABLE", "ENABLED", "ON"]], "Input"=w850, "Command"=w849, "Driver Name"=w855, "Error Code"=w854) -> ("Choice"=w851:string, "Error Out"=w853:errorcluster)  [unwired: 8 in]
                  n227 = call "MLLF_WriteToBuffer.vi"("String"=w851, "error in"=w853, "DriverConnect in"=w852) -> ("error out"=w862:T15, "DriverConnect out"=w861:T1)  [unwired: 5 in]
                  n228 = call "AgilentDMM_ESR_check.vi"("Driver Name"=w855, "Error Code"=w854, "Model"=w858, "error in"=w862, "DriverConnect in"=w861) -> ("error out"=w859:T15)  [unwired: 5 in, 1 out]
                }
                frame "SND", "Sound" {
                  # "sound"
                  # "sound=off"
                  n229 = call "MLLF_ParameterSelect.vi"("Command to equipment"=string[] ["SYST:BEEP:STAT OFF", "SYST:BEEP:STAT ON", "SYST:BEEP"] ("Names"), "Names"=string[][] [["0", "DIS", "DISABLED", "DISABLE", "OFF"], ["1", "EN", "ENABLE", "ENABLED", "ON"], [" ", "", "", "", ""]], "Input"=w864, "Command"=w863, "Driver Name"=w871, "Error Code"=w872) -> ("Choice"=w867:string, "Error Out"=w869:errorcluster)  [unwired: 8 in]
                  n230 = call "MLLF_WriteToBuffer.vi"("String"=w867, "error in"=w869, "DriverConnect in"=w868) -> ("error out"=w874:T15, "DriverConnect out"=w873:T1)  [unwired: 5 in]
                  n231 = call "AgilentDMM_ESR_check.vi"("Driver Name"=w871, "Error Code"=w872, "Model"=w875, "error in"=w874, "DriverConnect in"=w873) -> ("error out"=w870:T15)  [unwired: 5 in, 1 out]
                }
              }
            }
            frame #2 {
            }
          }
        }
        frame "get" {
          n232 = flat-sequence {
            tunnel: w898 -> [w909]
            tunnel: w899 -> [w910]
            tunnel: w900 -> [w911]
            tunnel: w888 -> [w902]
            tunnel: [w902] -> w897
            tunnel: [w911] -> w896
            tunnel: [w910] -> w895
            tunnel: [w907] -> w894
            tunnel: [w908] -> w893
            tunnel: [w906] -> w892
            tunnel: [w903] -> w891
            tunnel: [w904] -> w890
            tunnel: [w909] -> w889
            tunnel: w887 -> [w905]
            tunnel: w897 -> [w925]
            tunnel: w896 -> [w923]
            tunnel: w895 -> [w922]
            tunnel: w894 -> [w919]
            tunnel: w893 -> [w918]
            tunnel: w892 -> [w917]
            tunnel: w891 -> [w916]
            tunnel: w890 -> [w915]
            tunnel: w889 -> [w912]
            tunnel: [w924] -> w886
            tunnel: [w921] -> w885
            tunnel: [w920] -> w884
            tunnel: [w914] -> w883
            tunnel: [w913] -> w882
            tunnel: [w1064] -> w901
            tunnel: w886 -> [w1064]
            tunnel: w885 -> [w1062]
            tunnel: w884 -> [w1061]
            tunnel: w883 -> [w1063]
            tunnel: w882 -> [w1060]
            tunnel: [w1059] -> w881
            tunnel: [w1058] -> w880
            frame #0 {
              n233 = Unbundle By Name(w902) -> ("Permanent data.Model"=w908:T8, "Permanent data.Connect"=w907:T1, "Permanent data.Func"=w906:T7)
              n234 = call "MLLF_CommandDelimeter.vi"("command with param"=w905) -> ("param 1"=w904:string, "command"=w903:string)  [unwired: 6 in, 3 out]
            }
            frame #1 {
              n235 = case shown="\"CONF\", \"CONFIG\", \"CONFIGURATION\"" w916 {
                selector: w916 -> [w927 _ _ _ _ _ _]
                tunnel: [w926 w931 w945 w977 w992 w1018 w1044] -> w921
                tunnel: w923 -> [_ _ w938 w976 w985 w1011 w1038]
                tunnel: [w930 w934 w947 w979 w994 w1020 w1046] -> w924
                tunnel: w925 -> [w930 w934 w947 w979 w994 w1020 w1046]
                tunnel: [w928 w932 w940 _ w987 w1013 _] -> w920
                tunnel: w919 -> [_ _ w946 w978 w993 w1019 w1045]
                tunnel: w922 -> [_ _ w937 w975 w984 w1010 w1037]
                tunnel: w915 -> [_ _ w941 w967 w988 w1014 w1040]
                tunnel: w918 -> [_ _ w936 w974 w983 w1009 w1036]
                tunnel: w917 -> [_ _ w935 w973 w982 _ _]
                tunnel: [_ _ _ TRUE ("use system decimal point (T)") _ _ TRUE ("use system decimal point (T)")] -> w914
                tunnel: [_ _ _ w965 _ _ w1034] -> w913
                tunnel: w912 -> [_ w931 _ _ _ _ _]
                frame "False", Default {
                  n236 = call "MLLF_UnknownCommand(SubVI).vi"("Unknown command"=w927) -> ("error out"=w926:errorcluster)  [unwired: 10 in]
                  n237 = Build Array(0.0 ("TimeOut")) -> (w928:dbl[])
                }
                frame "TIMEOUT" {
                  n238 = Unbundle By Name(w934) -> ("Permanent data.Connect.InterfaceSettings.TMO, ms"=w933:i32)
                  n239 = Build Array(w933) -> (w932:i32[])
                }
                frame "READ" {
                  n240 = Decimal String To Number(string=w941) -> (number=w942:i32)  [unwired: 2 in, 1 out]
                  n241 = In Range and Coerce(upper limit=100, x=w942, lower limit=1) -> (coerced(x)=w939:i32)  [unwired: 1 out]
                  n242 = for {
                    N: w939 -> [_]
                    tunnel: [w959] -> w940 mode=indexing
                    tunnel: w946 -> [w958]
                    tunnel: [w953] -> w945
                    tunnel: w938 -> [w952]
                    tunnel: w937 -> [w951]
                    tunnel: w936 -> [w950]
                    tunnel: w935 -> [w948]
                    stop <- w953 stop-if-true
                    n243 = case shown="\"VDC\", Default" w948 {
                      tunnel: [1.0 ("Delay Time (s)") 0.05 ("Delay Time (s)")] -> w949
                      frame "F" {
                      }
                      frame "VDC", Default {
                      }
                    }
                    n244 = call "MLLF_WriteToBufferWithDelay.vi"("Delay Time ( 0,05 s)"=w949, "Command"="READ? " ("String"), "DriverConnect in"=w958) -> ("Error Out"=w962:errorcluster, "DriverConnect out"=w961:T1)  [unwired: 7 in]
                    n245 = call "MLLF_ReadBuffer.vi"("Error In"=w962, "DriverConnect in"=w961) -> ("Error Out"=w955:errorcluster, "DriverConnect out"=w954:T1, "String"=w957:string)  [unwired: 6 in]
                    n246 = call "AgilentDMM_ESR_check.vi"("Driver Name"=w951, "Error Code"=w952, "Model"=w950, "error in"=w955, "DriverConnect in"=w954) -> ("error out"=w953:T15)  [unwired: 5 in, 1 out]
                    n247 = Fract/Exp String To Number(use system decimal point (T)=FALSE, string=w957) -> (number=w959:dbl)  [unwired: 2 in, 1 out]
                  }
                }
                frame "SCPI" {
                  n248 = case shown="\"VDC\", Default" w973 {
                    tunnel: [1.0 ("Delay Time (s)") 0.05 ("Delay Time (s)")] -> w968
                    frame "F" {
                    }
                    frame "VDC", Default {
                    }
                  }
                  n249 = call "MLLF_WriteToBufferWithDelay.vi"("Delay Time ( 0,05 s)"=w968, "Command"=w967, "DriverConnect in"=w978) -> ("Error Out"=w972:errorcluster, "DriverConnect out"=w971:T1)  [unwired: 7 in]
                  n250 = call "MLLF_ReadBuffer.vi"("Error In"=w972, "DriverConnect in"=w971) -> ("Error Out"=w970:errorcluster, "DriverConnect out"=w969:T1, "String"=w965:string)  [unwired: 6 in]
                  n251 = call "AgilentDMM_ESR_check.vi"("Driver Name"=w975, "Error Code"=w976, "Model"=w974, "error in"=w970, "DriverConnect in"=w969) -> ("error out"=w977:T15)  [unwired: 5 in, 1 out]
                }
                frame "SelfTest" {
                  n252 = Decimal String To Number(string=w988) -> (number=w989:i32)  [unwired: 2 in, 1 out]
                  n253 = In Range and Coerce(upper limit=100, x=w989, lower limit=1) -> (coerced(x)=w986:i32)  [unwired: 1 out]
                  n254 = for {
                    N: w986 -> [_]
                    tunnel: [w1006] -> w987 mode=indexing
                    tunnel: w993 -> [w1005]
                    tunnel: [w1000] -> w992
                    tunnel: w985 -> [w999]
                    tunnel: w984 -> [w998]
                    tunnel: w983 -> [w997]
                    tunnel: w982 -> [_]
                    stop <- w1000 stop-if-true
                    n255 = call "MLLF_WriteToBufferWithDelay.vi"("Command"="*TST? " ("String"), "DriverConnect in"=w1005) -> ("Error Out"=w996:errorcluster, "DriverConnect out"=w1008:T1)  [unwired: 8 in]
                    n256 = call "Time Delay"("error in (no error)"=w996) -> ("error out"=w995:errorcluster)  [unwired: 10 in]
                    n257 = call "MLLF_ReadBuffer.vi"("Error In"=w995, "DriverConnect in"=w1008) -> ("Error Out"=w1002:errorcluster, "DriverConnect out"=w1001:T1, "String"=w1004:string)  [unwired: 6 in]
                    n258 = call "AgilentDMM_ESR_check.vi"("Driver Name"=w998, "Error Code"=w999, "Model"=w997, "error in"=w1002, "DriverConnect in"=w1001) -> ("error out"=w1000:T15)  [unwired: 5 in, 1 out]
                    n259 = Fract/Exp String To Number(use system decimal point (T)=FALSE, string=w1004) -> (number=w1006:dbl)  [unwired: 2 in, 1 out]
                  }
                }
                frame "FETCH" {
                  n260 = Decimal String To Number(string=w1014) -> (number=w1015:i32)  [unwired: 2 in, 1 out]
                  n261 = In Range and Coerce(upper limit=100, x=w1015, lower limit=1) -> (coerced(x)=w1012:i32)  [unwired: 1 out]
                  n262 = for {
                    N: w1012 -> [_]
                    tunnel: [w1030] -> w1013 mode=indexing
                    tunnel: w1019 -> [w1029]
                    tunnel: [w1024] -> w1018
                    tunnel: w1011 -> [w1023]
                    tunnel: w1010 -> [w1022]
                    tunnel: w1009 -> [w1021]
                    stop <- w1024 stop-if-true
                    n263 = call "MLLF_WriteToBuffer.vi"("String"="FETC? ", "DriverConnect in"=w1029) -> ("error out"=w1033:T15, "DriverConnect out"=w1032:T1)  [unwired: 6 in]
                    n264 = call "MLLF_ReadBuffer.vi"("Error In"=w1033, "DriverConnect in"=w1032) -> ("Error Out"=w1026:errorcluster, "DriverConnect out"=w1025:T1, "String"=w1028:string)  [unwired: 6 in]
                    n265 = call "AgilentDMM_ESR_check.vi"("Driver Name"=w1022, "Error Code"=w1023, "Model"=w1021, "error in"=w1026, "DriverConnect in"=w1025) -> ("error out"=w1024:T15)  [unwired: 5 in, 1 out]
                    n266 = Fract/Exp String To Number(use system decimal point (T)=FALSE, string=w1028) -> (number=w1030:dbl)  [unwired: 2 in, 1 out]
                  }
                }
                frame "CONF", "CONFIG", "CONFIGURATION" {
                  n267 = Decimal String To Number(string=w1040) -> (number=w1041:i32)  [unwired: 2 in, 1 out]
                  n268 = In Range and Coerce(upper limit=100, x=w1041, lower limit=1) -> (coerced(x)=w1039:i32)  [unwired: 1 out]
                  n269 = for {
                    N: w1039 -> [_]
                    tunnel: w1045 -> [w1055]
                    tunnel: [w1051] -> w1044
                    tunnel: w1038 -> [w1050]
                    tunnel: w1037 -> [w1049]
                    tunnel: w1036 -> [w1048]
                    tunnel: [w1047] -> w1034
                    stop <- w1051 stop-if-true
                    n270 = call "MLLF_WriteToBuffer.vi"("String"="CONFigure? ", "DriverConnect in"=w1055) -> ("error out"=w1057:T15, "DriverConnect out"=w1056:T1)  [unwired: 6 in]
                    n271 = call "MLLF_ReadBuffer.vi"("Error In"=w1057, "DriverConnect in"=w1056) -> ("Error Out"=w1053:errorcluster, "DriverConnect out"=w1052:T1, "String"=w1047:string)  [unwired: 6 in]
                    n272 = call "AgilentDMM_ESR_check.vi"("Driver Name"=w1049, "Error Code"=w1050, "Model"=w1048, "error in"=w1053, "DriverConnect in"=w1052) -> ("error out"=w1051:T15)  [unwired: 5 in, 1 out]
                  }
                }
              }
            }
            frame #2 {
              n273 = case shown="False" w1063 {
                tunnel: w1062 -> [w1069 w1070]
                tunnel: w1061 -> [w1068 _]
                tunnel: [w1066 w1070] -> w1059
                tunnel: [w1065 w1071] -> w1058
                tunnel: w1060 -> [_ w1071]
                frame False {
                  n274 = call "MLLF_FormatOutputValueWithUnits.vi"("Format"="%.;%^#_8e" ("format string"), "error in"=w1069, "ValuesIn"=w1068) -> ("error out"=w1066:T15, "Result string"=w1065:T16)  [unwired: 7 in]
                }
                frame True {
                }
              }
            }
          }
        }
        frame "close" {
          n275 = Unbundle By Name(w1073) -> ("Permanent data.Connect.OpenedSession"=w1075:T3)
          n276 = VISA Close(VISA resource name=w1075) -> (error out=w1074:errorcluster)  [unwired: 1 in]
        }
      }
    }
    frame Error {
    }
  }
  n277 = local write "Settings"(w1) -> ()
  n278 = flat-sequence {
    tunnel: [w1087] -> w2
    tunnel: [w1086] -> w4
    tunnel: w7 -> [w1085]
    tunnel: w5 -> [w1084]
    tunnel: w6 -> [w1080]
    tunnel: [w1082] -> w3
    frame #0 {
      # "driver out"
      n279 = Unbundle By Name(w1080) -> ("Permanent data"=w1079:T17)
      n280 = To Variant(anything=w1079) -> (Variant=w1081:variant)
      n281 = Bundle By Name(cluster=w1080, "Saved Data"=w1081) -> (w1082:T9)
      n282 = call "MLLF_SaveLastSettingUtility.vi"("error in"=w1084, "Saved Data"=w1081) -> ("error out"=w1083:T15)  [unwired: 8 in, 1 out]
      n283 = call "MCF_Output.vi"("Error In"=w1083, "Input"=w1085) -> ("Error Out"=w1086:errorcluster, "Output"=w1087:string)  [unwired: 8 in]
    }
  }
  n284 = local write "Settings"(w3) -> ()
  "error out" <- w4
  "Response" <- w2
